vi "Neilpad.vi"(10 "Separator":string="\t", 11 "Input String Array":string[](array[string])) -> (3 "Output String":string)   [LabVIEW 2015]
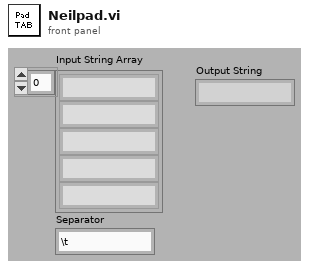
[diagram p1: front panel]
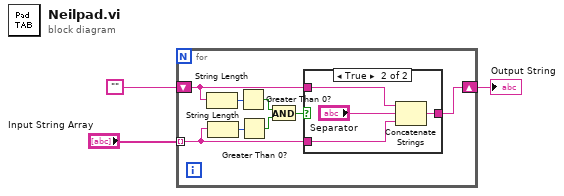
[diagram p0: block diagram]
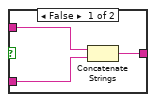
[diagram p2: hidden frame]
diagram:
  n1 = for {
    tunnel: "Input String Array" -> [w5] mode=indexing
    shift-right: [w4] -> w1
    shift-left: "" -> [w6]
    n2 = String Length(string=w6) -> (length=w11:i32)
    n3 = String Length(string=w5) -> (length=w10:i32)
    n4 = Greater Than 0?(x=w11) -> (x > 0?=w8:bool)
    n5 = Greater Than 0?(x=w10) -> (x > 0?=w9:bool)
    n6 = And(x=w8, y=w9) -> (x .and. y?=w7:bool)
    n7 = case shown="True" w7 {
      tunnel: w6 -> [w13 w17]
      tunnel: [w14 w18] -> w4
      tunnel: w5 -> [w12 w16]
      frame False {
        n8 = Concatenate Strings(w13, w12) -> (w14:string)
      }
      frame True {
        n9 = Concatenate Strings(w17, "Separator", w16) -> (w18:string)
      }
    }
  }
  "Output String" <- w1
